vi "Processing Arrays with For Loops.vi"() -> ()   [LabVIEW 2023]
panel:
  out "Output Array":dbl[](array[numeric])
  out "Current Value":dbl
  in  "Input Array":dbl[](array[numeric])
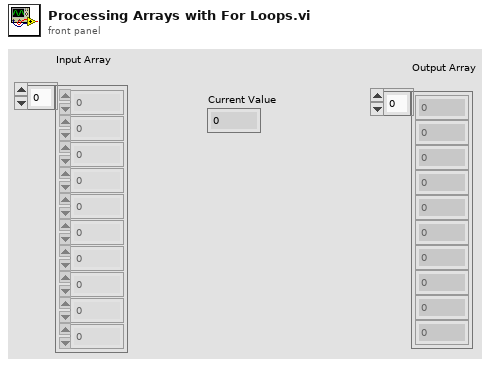
[diagram p1: front panel]
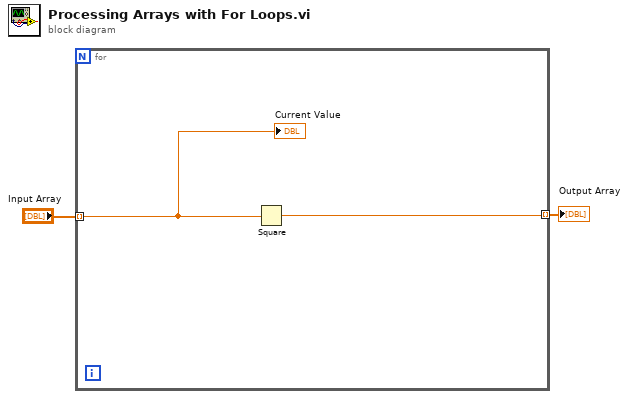
[diagram p0: block diagram]
diagram:
  n1 = for {
    tunnel: "Input Array" -> [w4] mode=indexing
    tunnel: [w3] -> w1 mode=indexing
    n2 = Square(x=w4) -> (x^2=w3:dbl)
    "Current Value" <- w4
  }
  "Output Array" <- w1
